vi "DS18x20 Temperature Sensor.vi"() -> ()   [LabVIEW 2014]
doc: "This example shows how to read temp data from DS18x20 sensor."
uses:
  QwaveSys_Interface/QwaveSys_Interface.lvlib
  PWS_ESP8266/PWS_ESP8266.lvlib
panel:
  in  "DS18x20":u8(ring)=15 items=["SPI#1/SS,(5)"=5, "SPI#2/MOSI,(13)"=13, "SPI#3/MISO,(12)"=12, "SPI#4/SCLK,(14)"=14, "UART#1/CS,(15)"=15, "UART#2/TXD,(1)"=1, "UART#3/RXD,(3)"=3, "UART#4/LED,(16)"=16, "FPROM_Btn,(0)"=0, "SDCard_CS,(4)"=4, "I2C-SDA/TXD1,(2)"=2, "ADC0,(17)"=17]
  # "Overview: Demonstrates how to read  DS18x20 sensor connected to digital pin.\nRequirements: LabVIEW Full Development System,Arduino Compatible Compiler for LabVIEW,Programmable Wireless Stamp (PWS) Library.\nInstructions:\n1. Wire a temperature sensor DS18x20 (This example using DS18b20) as specified below where the data pin is wired to the specified Digital Pin (GPIO15) below.\n2.  If this example has been loaded from the Arduino Compatible Compiler for LabVIEW, simply select Compile and Download.  Otherwise, open Tools>Arduino Compatible Compiler for LabVIEW in LabVIEW, then select File>Load VI, and select this VI and then Compile and Download.\n3. Open \"Serial Monitor\" by select \"Tools>Serial Monitor\" and select baud rate to 9600.\n4. Observe the logged data being print out on serial port monitor."
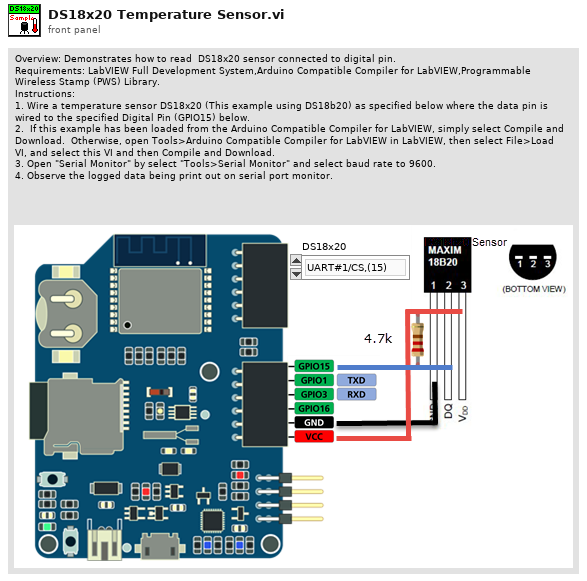
[diagram p1: front panel]
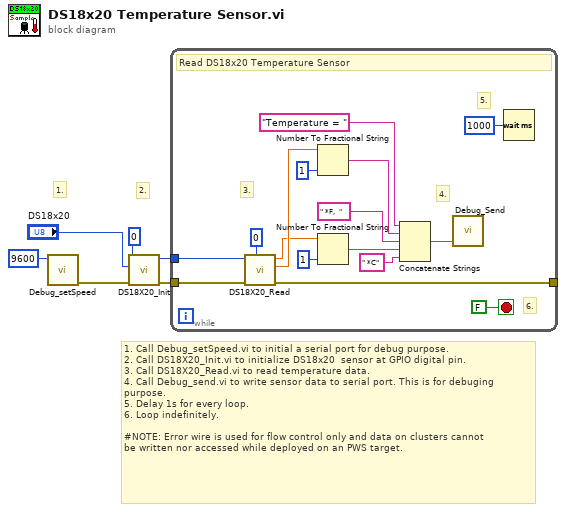
[diagram p0: block diagram]
diagram:
  # "1. Call Debug_setSpeed.vi to initial a serial port for debug purpose.\n2. Call DS18X20_Init.vi to initialize DS18x20  sensor at GPIO digital pin. \n3. Call DS18X20_Read.vi to read temperature data.\n4. Call Debug_send.vi to write sensor data to serial port. This is for debuging purpose.\n5. Delay 1s for every loop.\n6. Loop indefinitely.\n\n#NOTE: Error wire is used for flow control only and data on clusters cannot\nbe written nor accessed while deployed on an PWS target."
  # "2."
  # "1."
  n1 = call "Debug_setSpeed.vi"("Speed"=u32 9600) -> ("error out"=w3:errorcluster)  [unwired: 10 in]
  n2 = call "DS18X20_Init.vi"("error in"=w3, "PIN"="DS18x20", "Interface (0-4)"=u8 0) -> ("error out"=w6:errorcluster, "Instance"=w5:u8)  [unwired: 7 in]
  n3 = while {
    tunnel: w6 -> [w22]
    tunnel: w5 -> [w10]
    tunnel: [w7] -> _
    stop <- FALSE stop-if-true
    # "6."
    # "5."
    # "4."
    # "3."
    # "Read DS18x20 Temperature Sensor"
    n4 = call "DS18X20_Read.vi"("Index"=i8 0, "error in (no error)"=w22, "Instance"=w10) -> ("error out"=w7:errorcluster, "F"=w16:dbl, "C"=w15:dbl)  [unwired: 6 in]
    n5 = Number To Fractional String(number=w16, precision (6)=i16 1) -> (F-format string=w20:string)  [unwired: 2 in]
    n6 = Number To Fractional String(number=w15, precision (6)=i16 1) -> (F-format string=w19:string)  [unwired: 2 in]
    n7 = Concatenate Strings("Temperature = " ("format string"), w20, " *F,  " ("format string"), w19, " *C" ("string")) -> (w8:string)
    n8 = call "Debug_Send.vi"("DATA"=w8) -> ()  [unwired: 11 in]
    n9 = Wait (ms)(milliseconds to wait=u32 1000) -> ()  [unwired: 1 out]
  }
